vi "LTVUnicycleCtrl_Calculate_ORIG.vi"(6 "RefAngularVelocity":dbl, 8 "RefLinearVelocity":dbl, 9 "RefPose":T2={"TRANSLATION"={"X"=0.0, "Y"=0.0}, "ROTATION"={"VALUE"=0.0, "COS"=1.0, "SIN"=0.0}} {"ROTATION"."SIN" format="%13.4f"; "ROTATION"."COS" format="%13.4f"; "ROTATION"."VALUE" format="%13.4f"; "TRANSLATION"."Y" format="%14.3f"; "TRANSLATION"."X" format="%14.3f"}, 10 "CurrentPose":T2={"TRANSLATION"={"X"=0.0, "Y"=0.0}, "ROTATION"={"VALUE"=0.0, "COS"=1.0, "SIN"=0.0}} {"ROTATION"."SIN" format="%13.4f"; "ROTATION"."COS" format="%13.4f"; "ROTATION"."VALUE" format="%13.4f"; "TRANSLATION"."Y" format="%14.3f"; "TRANSLATION"."X" format="%14.3f"}, 11 "in LTV_UNICYCLE_CONTROLLER":T5={"m_A"=[], "m_B"=[], "m_Q"=[], "m_R"=[], "States"=0, "Inputs"=0, "PoseError"={"TRANSLATION"={"X"=0.0, "Y"=0.0}, "ROTATION"={"VALUE"=0.0, "COS"=1.0, "SIN"=0.0}}, "PoseTolerance"={"TRANSLATION"={"X"=0.0, "Y"=0.0}, "ROTATION"={"VALUE"=0.0, "COS"=1.0, "SIN"=0.0}}, "Dt"=0.02, "Enabled"=FALSE, "savedLQR_K"={"Table Xs"=[], "Table Ys"=[], "MinX"=0.0, "MaxX"=0.0, "ItemCount"=0, "Rows"=0, "Columns"=0}} {"PoseTolerance"."ROTATION"."SIN" format="%13.4f"; "PoseTolerance"."ROTATION"."COS" format="%13.4f"; "PoseTolerance"."ROTATION"."VALUE" format="%13.4f"; "PoseTolerance"."TRANSLATION"."Y" format="%14.3f"; "PoseTolerance"."TRANSLATION"."X" format="%14.3f"; "PoseError"."ROTATION"."SIN" format="%13.4f"; "PoseError"."ROTATION"."COS" format="%13.4f"; "PoseError"."ROTATION"."VALUE" format="%13.4f"; "PoseError"."TRANSLATION"."Y" format="%14.3f"; "PoseError"."TRANSLATION"."X" format="%14.3f"}) -> (0 "Error":bool, 2 "ChassisSpeeds":T1 {"vOmega" format="%10.3f"; "vY" format="%10.3f"; "vX" format="%10.3f"}, 3 "out LTV_UNICYCLE_CONTROLLER":T5={"m_A"=[], "m_B"=[], "m_Q"=[], "m_R"=[], "States"=0, "Inputs"=0, "PoseError"={"TRANSLATION"={"X"=0.0, "Y"=0.0}, "ROTATION"={"VALUE"=0.0, "COS"=1.0, "SIN"=0.0}}, "PoseTolerance"={"TRANSLATION"={"X"=0.0, "Y"=0.0}, "ROTATION"={"VALUE"=0.0, "COS"=1.0, "SIN"=0.0}}, "Dt"=0.02, "Enabled"=FALSE, "savedLQR_K"={"Table Xs"=[], "Table Ys"=[], "MinX"=0.0, "MaxX"=0.0, "ItemCount"=0, "Rows"=0, "Columns"=0}} {"PoseTolerance"."ROTATION"."SIN" format="%13.4f"; "PoseTolerance"."ROTATION"."COS" format="%13.4f"; "PoseTolerance"."ROTATION"."VALUE" format="%13.4f"; "PoseTolerance"."TRANSLATION"."Y" format="%14.3f"; "PoseTolerance"."TRANSLATION"."X" format="%14.3f"; "PoseError"."ROTATION"."SIN" format="%13.4f"; "PoseError"."ROTATION"."COS" format="%13.4f"; "PoseError"."ROTATION"."VALUE" format="%13.4f"; "PoseError"."TRANSLATION"."Y" format="%14.3f"; "PoseError"."TRANSLATION"."X" format="%14.3f"})   [LabVIEW 2019, in "Trajectory_Library.lvlib"]
doc: "Create implicit model follower\n\nInputs:\n - A < states, states > -- Continuous system matrix of the plant being controlled.\n - B < states, inputs > -- Continuous input matrix of the plant being controlled.\n - A_Ref < states, states > -- Continuous system matrix whose dymanics should be followed.\n - B_Ref < states, inputs > -- Continuous input matrix x whose dymanics should be followed.\n\nOutputs:\n - Error -- If TRUE, an error occured."
uses:
  Trajectory_Library.lvlib
  TypeDef/LTV_UNICYCLE_CONTROLLER_STATE_ENUM.ctl
  <vilib>/Analysis/NI_AALBase.lvlib
  <vilib>/Analysis/baseanly.llb/Real A x B.vi
  <vilib>/Analysis/Matrix/Datatypes/RealMatrix.ctl
  <vilib>/Analysis/Matrix/NI_Matrix.lvlib
  TypeDef/LTV_UNICYCLE_CONTROLLER.ctl
  TRANSLATION2D.ctl
  ROTATION2D.ctl
  POSE2D.ctl
  CHASSIS_SPEEDS.ctl
  TypeDef/FUNCTION_GENERATOR_MATRIX.ctl
panel:
  # "<States,States>"
  # "<States,Inputs>"
  # "<States, States>"
  # "<Inputs, Inputs>"
  # "<States,States>"
  # "<States,Inputs>"
  # "<States, States>"
  # "<Inputs, Inputs>"
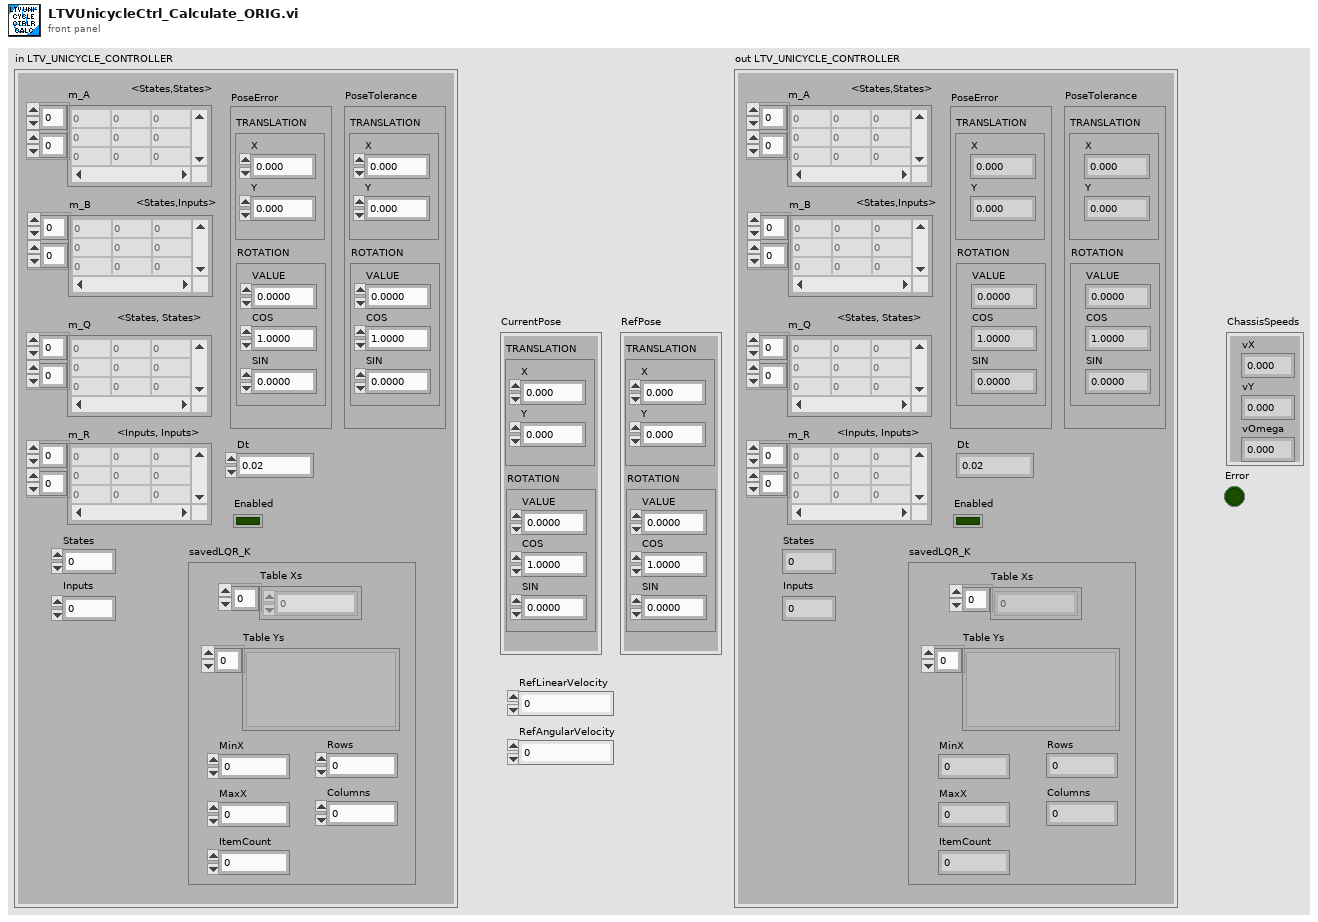
[diagram p1: front panel]
types:
  T1 = typedef "Trajectory_Library.lvlib/CHASSIS_SPEEDS.ctl" = cluster{"vX":dbl, "vY":dbl, "vOmega":dbl}
  T2 = typedef "Trajectory_Library.lvlib/POSE2D.ctl" = cluster{"TRANSLATION":T3, "ROTATION":T4}
  T3 = typedef "Trajectory_Library.lvlib/TRANSLATION2D.ctl" = cluster{"X":dbl, "Y":dbl}
  T4 = typedef "Trajectory_Library.lvlib/ROTATION2D.ctl" = cluster{"VALUE":dbl, "COS":dbl, "SIN":dbl}
  T5 = typedef "Trajectory_Library.lvlib/LTV_UNICYCLE_CONTROLLER.ctl" = cluster{"m_A":T6, "m_B":T6, "m_Q":T6, "m_R":T6, "States":i32, "Inputs":i32, "PoseError":T2, "PoseTolerance":T2, "Dt":dbl, "Enabled":bool, "savedLQR_K":T7}
  T6 = typedef "NI_Matrix.lvlib/RealMatrix.ctl" = dbl[][]
  T7 = typedef "Trajectory_Library.lvlib/FUNCTION_GENERATOR_MATRIX.ctl" = cluster{"Table Xs":dbl[], "Table Ys":variant[], "MinX":dbl, "MaxX":dbl, "ItemCount":i32, "Rows":i32, "Columns":i32}
  T8 = typedef "Trajectory_Library.lvlib/LTV_UNICYCLE_CONTROLLER_STATE_ENUM.ctl" = enum16{"X", "Y", "HEADING"}
  T9 = typedef "Trajectory_Library.lvlib/LINEAR_QUADRATIC_REGULATOR.ctl" = cluster{"m_r":T6, "m_U":T6, "m_K":T6, "States":i32, "Inputs":i32}
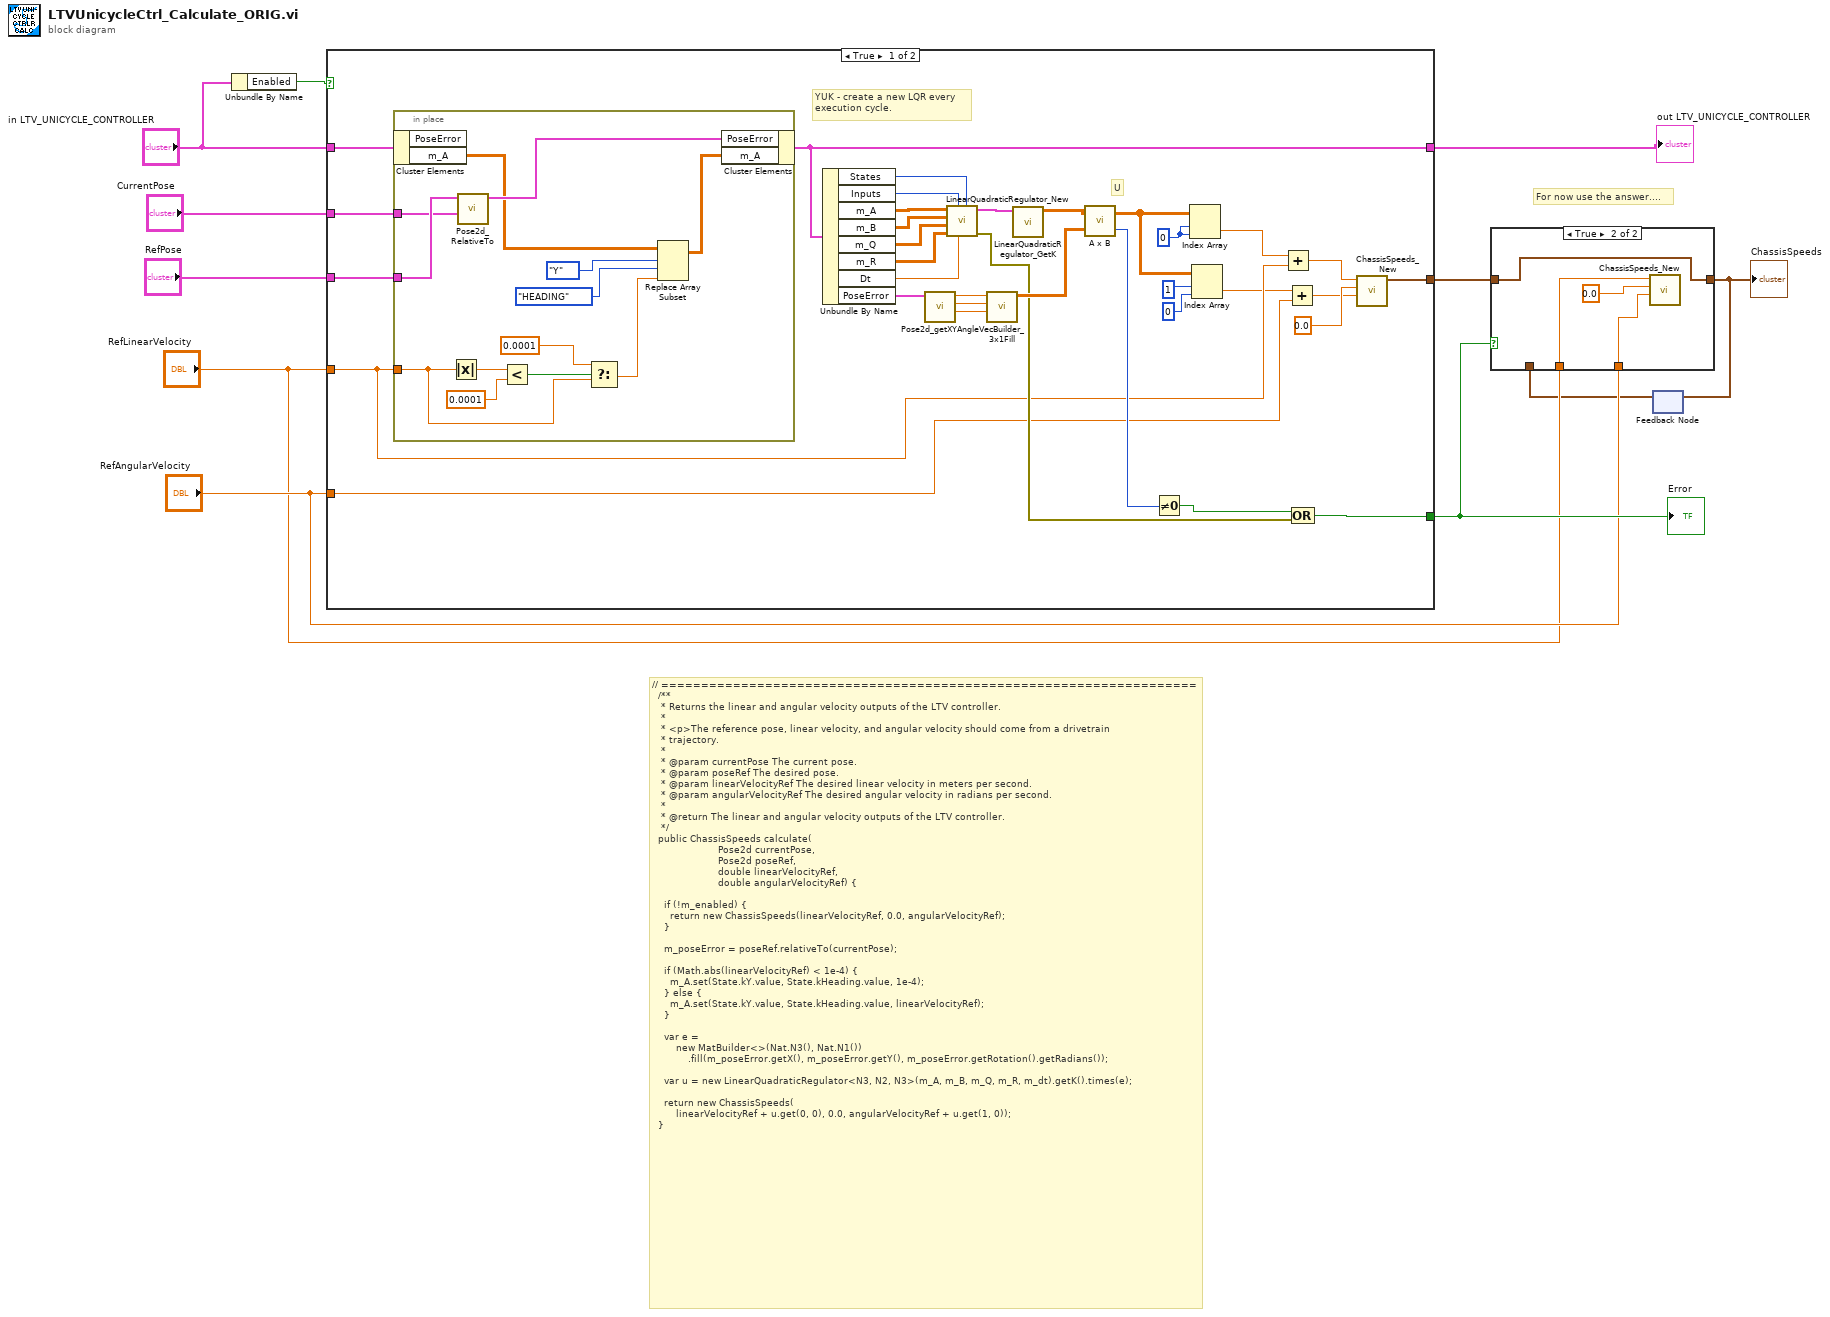
[diagram p0: block diagram]
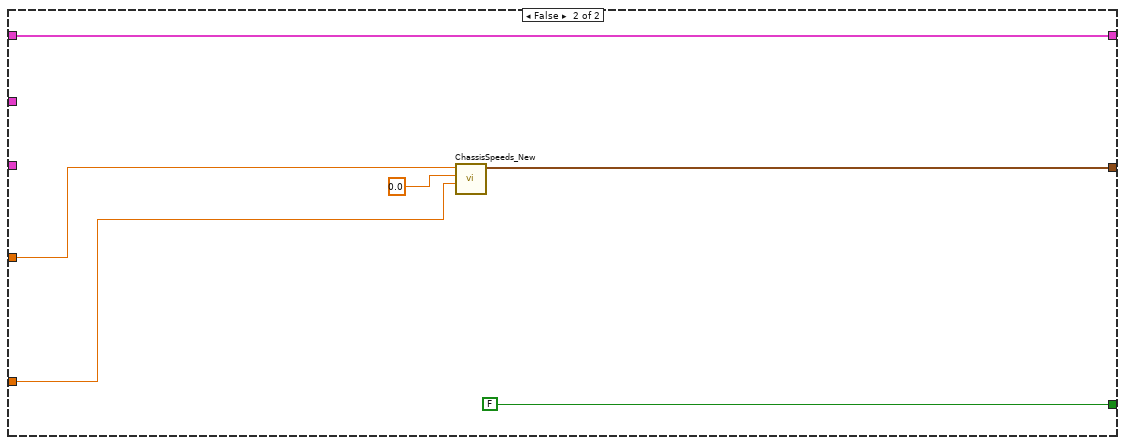
[diagram p3: hidden frame]
diagram:
  # "For now use the answer...."
  # "// ===================================================================\n  /**\n   * Returns the linear and angular velocity outputs of the LTV controller.\n   *\n   * <p>The reference pose, linear velocity, and angular velocity should come from a drivetrain\n   * trajectory.\n   *\n   * @param currentPose The current pose.\n   * @param poseRef The desired pose.\n   * @param linearVelocityRef The desired linear velocity in meters per second.\n   * @param angularVelocityRef The desired angular velocity in radians per second.\n   *\n   * @return The linear and angular velocity outputs of the LTV controller.\n   */\n  public ChassisSpeeds calculate(\n      \t               Pose2d currentPose, \n       \t              Pose2d poseRef, \n\t                     double linearVelocityRef, \n\t                     double angularVelocityRef) {\n\n    if (!m_enabled) {\n      return new ChassisSpeeds(linearVelocityRef, 0.0, angularVelocityRef);\n    }\n\n    m_poseError = poseRef.relativeTo(currentPose);\n\n    if (Math.abs(linearVelocityRef) < 1e-4) {\n      m_A.set(State.kY.value, State.kHeading.value, 1e-4);\n    } else {\n      m_A.set(State.kY.value, State.kHeading.value, linearVelocityRef);\n    }\n\n    var e =\n        new MatBuilder<>(Nat.N3(), Nat.N1())\n            .fill(m_poseError.getX(), m_poseError.getY(), m_poseError.getRotation().getRadians());\n\n    var u = new LinearQuadraticRegulator<N3, N2, N3>(m_A, m_B, m_Q, m_R, m_dt).getK().times(e);\n\n    return new ChassisSpeeds(\n        linearVelocityRef + u.get(0, 0), 0.0, angularVelocityRef + u.get(1, 0));\n  }"
  n1 = Unbundle By Name("in LTV_UNICYCLE_CONTROLLER") -> ("Enabled"=w11:bool)
  n2 = case shown="True" w11 {
    tunnel: "in LTV_UNICYCLE_CONTROLLER" -> [w45 w64]
    tunnel: [w42 w64] -> w9
    tunnel: [w12 FALSE] -> w6
    tunnel: [w24 w62] -> w5
    tunnel: "RefLinearVelocity" -> [w20 w61]
    tunnel: "RefAngularVelocity" -> [w19 w60]
    tunnel: "RefPose" -> [w44 _]
    tunnel: "CurrentPose" -> [w43 _]
    frame True {
      w18 = 0 ("index (row)")
      # "U"
      # "YUK - create a new LQR every\nexecution cycle."
      n3 = in-place {
        in-place-border: w44 -> [w58]
        in-place-border: w43 -> [w57]
        in-place-border: w20 -> [w47]
        n4 = in-place-cluster #1(w45) -> ("m_A"=w53:T6)  [unwired: 1 out]
        n5 = Absolute Value(x=w47) -> (abs(x)=w55:dbl)
        n6 = call "Pose2d_RelativeTo.vi"("other POSE"=w57, "in POSE"=w58) -> ("out POSE"=w56:T2)  [unwired: 9 in]
        n7 = Less?(x=w55, y=0.0001) -> (x < y?=w49:bool)
        n8 = Select(t=0.0001, s=w49, f=w47) -> (s? t:f=w46:dbl)
        n9 = Replace Array Subset(array=w53, new element=w46, index (row)=LTV_UNICYCLE_CONTROLLER_STATE_ENUM."Y" ("LTV_UNICYCLE_CONTROLLER_STATE"), index (col)=LTV_UNICYCLE_CONTROLLER_STATE_ENUM."HEADING" ("LTV_UNICYCLE_CONTROLLER_STATE")) -> (w52:T6)
        n10 = in-place-cluster #1("PoseError"=w56, "m_A"=w52) -> (w42:T5)
      }
      n11 = Unbundle By Name(w42) -> ("States"=w41:i32, "Inputs"=w40:i32, "m_A"=w39:T6, "m_B"=w38:T6, "m_Q"=w37:T6, "m_R"=w36:T6, "Dt"=w35:dbl, "PoseError"=w33:T2)
      n12 = call "Pose2d_getXYAngle.vi"("in POSE"=w33) -> ("Angle"=w30:dbl, "Y"=w31:dbl, "X"=w32:dbl)  [unwired: 8 in]
      n13 = call "LinearQuadraticRegulator_New.vi"("States"=w41, "dt_Seconds"=w35, "Inputs"=w40, "R"=w36, "Q"=w37, "B"=w38, "A"=w39) -> ("Error"=w27:errorcluster, "LinearQuadraticRegulator"=w34:T9)  [unwired: 3 in]
      n14 = call "VecBuilder_3x1Fill.vi"("R2"=w30, "R1"=w31, "R0"=w32) -> ("output matrix"=w28:T6)  [unwired: 8 in]
      n15 = call "LinearQuadraticRegulator_GetK.vi"("in LinearQuadraticRegulator"=w34) -> ("K"=w29:T6)  [unwired: 10 in]
      n16 = call-poly <vilib>:"A x B.vi"("B"=w28, "A"=w29) -> ("error"=w26:i32, "A x B"=w15:T6)
      n17 = Not Equal To 0?(x=w26) -> (x != 0?=w25:bool)
      n18 = Index Array(array=w15, index (row)=w18, index (col)=w18) -> (element=w14:dbl)
      n19 = Index Array(array=w15, index (row)=1, index (col)=0 ("index (row)")) -> (element=w13:dbl)
      n20 = Add(x=w14, y=w20) -> (x+y=w22:dbl)
      n21 = Add(x=w13, y=w19) -> (x+y=w21:dbl)
      n22 = Compound Arithmetic op=OR(w25, w27) -> (w12:bool)
      n23 = call "ChassisSpeeds_New.vi"("vAngular"=w21, "vY"=0.0, "vX"=w22) -> ("CHASSIS"=w24:T1)  [unwired: 8 in]
    }
    frame False {
      n24 = call "ChassisSpeeds_New.vi"("vAngular"=w60, "vY"=0.0, "vX"=w61) -> ("CHASSIS"=w62:T1)  [unwired: 8 in]
    }
  }
  "out LTV_UNICYCLE_CONTROLLER" <- w9
  "Error" <- w6
  n25 = feedback #2() -> (w1:T1)  [unwired: 1 in]
  n26 = case shown="True" w6 {
    tunnel: w5 -> [w65 w66]
    tunnel: [w65 w66] -> w2
    tunnel: "RefAngularVelocity" -> [_ w68]
    tunnel: "RefLinearVelocity" -> [_ w67]
    tunnel: w1 -> [_ _]
    frame False {
    }
    frame True {
      n27 = call "ChassisSpeeds_New.vi"("vAngular"=w68, "vY"=0.0, "vX"=w67) -> ()  [unwired: 8 in, 1 out]
    }
  }
  "ChassisSpeeds" <- w2
  n28 = feedback-in #2(w2) -> ()
